vi "velleman-close.vi"(1 "isActive":bool) -> (0 "error":bool)   [LabVIEW 2017]
uses:
  other/velleman/K8055D.dll
panel:
  out "error out":errorcluster
  out "open":i32
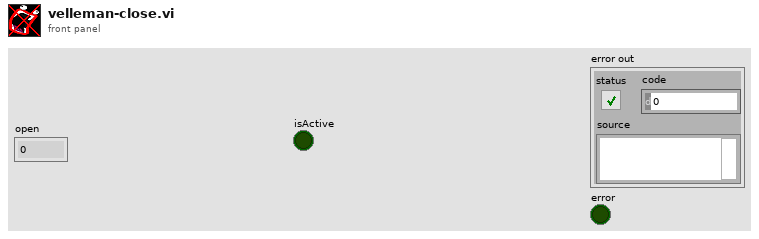
[diagram p1: front panel]
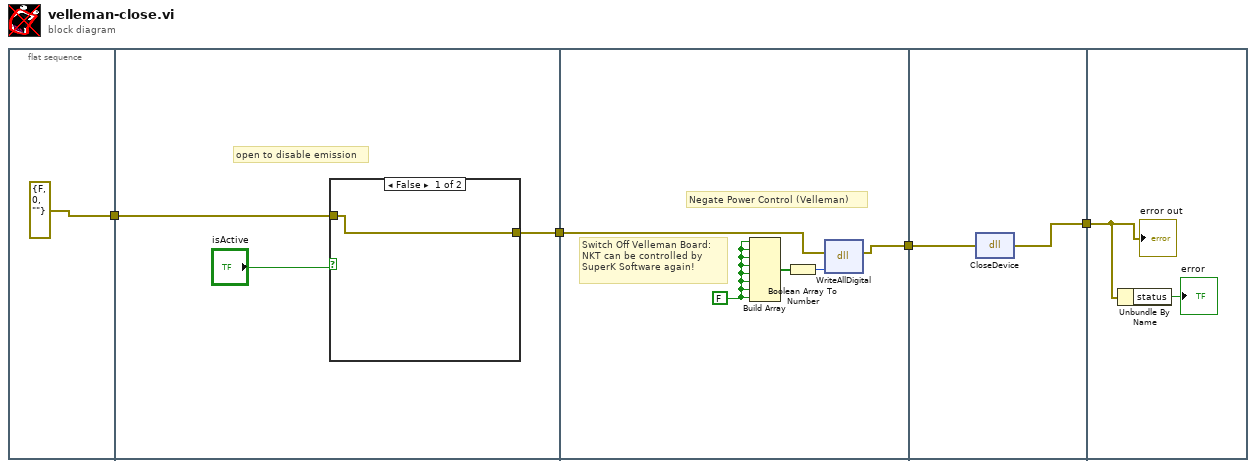
[diagram p0: block diagram]
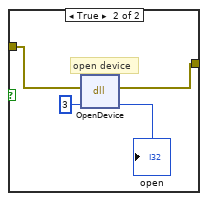
[diagram p2: hidden frame]
diagram:
  n1 = flat-sequence {
    tunnel: [errorcluster {"status"=FALSE, "code"=0, "source"=""} ("error in (no error)")] -> w2
    tunnel: [w6] -> w4
    tunnel: w2 -> [w7]
    tunnel: w4 -> [w15]
    tunnel: [w14] -> w3
    tunnel: w3 -> [w20]
    tunnel: [w19] -> w1
    tunnel: w1 -> [w22]
    frame #0 {
    }
    frame #1 {
      # "open to disable emission"
      n2 = case shown="False" "isActive" {
        tunnel: w7 -> [w9 w11]
        tunnel: [w9 w10] -> w6
        frame False {
        }
        frame True {
          # "open device"
          n3 = dll-call lib="D:/Programs/LabView/labview-plem/other/velleman/K8055D.dll" fn="OpenDevice"(error in=w11, 3) -> (error out=w10:errorcluster, →"open":i32)  [unwired: 3 in, 1 out]
        }
      }
    }
    frame #2 {
      w16 = FALSE ("Power Control")
      # "Negate Power Control (Velleman)"
      # "Switch Off Velleman Board:\nNKT can be controlled by\nSuperK Software again!"
      n4 = Build Array(w16, w16, w16, w16, w16, w16, w16, w16) -> (w18:bool[])
      n5 = Boolean Array To Number(Boolean array=w18) -> (number=w17:u32)
      n6 = dll-call lib="D:/Programs/LabView/labview-plem/other/velleman/K8055D.dll" fn="WriteAllDigital"(error in=w15, w17) -> (error out=w14:errorcluster)  [unwired: 4 in, 1 out]
    }
    frame #3 {
      n7 = dll-call lib="D:/Programs/LabView/labview-plem/other/velleman/K8055D.dll" fn="CloseDevice" label="Close Velleman Board"(error in=w20) -> (error out=w19:errorcluster)  [unwired: 3 in, 1 out]
    }
    frame #4 {
      n8 = Unbundle By Name(w22) -> ("status"=→"error":bool)
      "error out" <- w22
    }
  }
